vi "MGI RWA Process Array Elements.vi"(5 "Read/Write Options":T1={"TS Fmt"="", "Int Fmt"="", "Delimiter"=","}, 7 "Format String (%#0.15f)":string="%#0.15f", 8 "Error In":errorcluster, 9 "Name In":string, 10 "Array Variant":variant, 11 "Queue In":refnum<queue>) -> (0 "Error Out":errorcluster, 1 "Data Out":string, 3 "Queue Out":refnum<queue>)   [LabVIEW 2024]
doc: "This VI was created for use with the Read/Write Anything VIs. It converts array elements of the cluster to strings to be written to file.\n\nAuthored by Robert C. Mortensen\nsupport@mooregoodideas.com\nwww.mooregoodideas.com\n\nCopyright (c) 2010, Moore Good Ideas, Inc.\n\nAll rights reserved.\n\nRedistribution and use in source and binary forms, with or without modification, are permitted provided that the following conditions are met:\n\n * Redistributions of source code must retain the above copyright notice, this list of conditions and the following disclaimer.\n * Redistributions in binary form must reproduce the above copyright notice, this list of conditions and the following disclaimer in the documentation and/or other materials provided with the distribution.\n * Neither the name of Moore Good Ideas, Inc. nor the names of its contributors may be used to endorse or promote products derived from this software without specific prior written permission.\n\nTHIS SOFTWARE IS PROVIDED BY THE COPYRIGHT HOLDERS AND CONTRIBUTORS \"AS IS\" AND ANY EXPRESS OR IMPLIED WARRANTIES, INCLUDING, BUT NOT LIMITED TO, THE IMPLIED WARRANTIES OF MERCHANTABILITY AND FITNESS FOR A PARTICULAR PURPOSE ARE DISCLAIMED. IN NO EVENT SHALL THE COPYRIGHT OWNER OR CONTRIBUTORS BE LIABLE FOR ANY DIRECT, INDIRECT, INCIDENTAL, SPECIAL, EXEMPLARY, OR CONSEQUENTIAL DAMAGES (INCLUDING, BUT NOT LIMITED TO, PROCUREMENT OF SUBSTITUTE GOODS OR SERVICES; LOSS OF USE, DATA, OR PROFITS; OR BUSINESS INTERRUPTION) HOWEVER CAUSED AND ON ANY THEORY OF LIABILITY, WHETHER IN CONTRACT, STRICT LIABILITY, OR TORT (INCLUDING NEGLIGENCE OR OTHERWISE) ARISING IN ANY WAY OUT OF THE USE OF THIS SOFTWARE, EVEN IF ADVISED OF THE POSSIBILITY OF SUCH DAMAGE."
uses:
  MGI RWA Options Cluster.ctl
  MGI RWA Convertion Direction Enum.ctl
  VariantType.lvlib
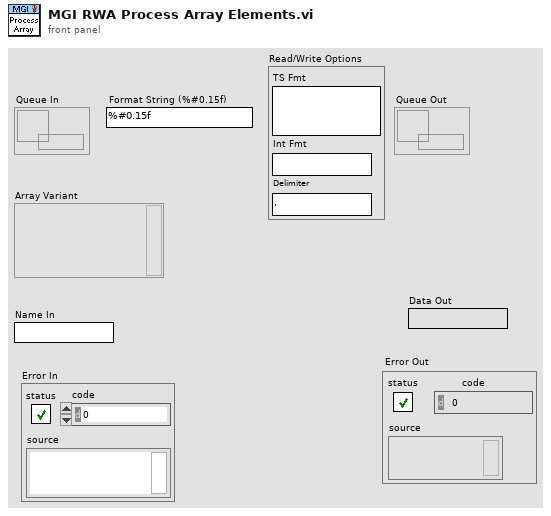
[diagram p1: front panel]
types:
  T1 = typedef "MGI RWA Options Cluster.ctl" = cluster{"TS Fmt":string, "Int Fmt":string, "Delimiter":string}
  T2 = typedef "VariantType.lvlib/Type.ctl" = enum8{"Invalid Type", "Void", "I8", "I16", "I32", "I64", "U8", "U16", "U32", "U64", "Single Float", "Double Float", "Extended Float", "Single Complex", "Double Complex", "Extended Complex", "Enum U8", "Enum U16", "Enum U32", "Enum U64", "Single Float With Unit", "Double Float With Unit", "Extended Float With Unit", "Single Complex with Unit", "Double Complex with Unit", "Extended Complex with Unit", "Boolean", "String", "Path", "Picture", "Tag", "Array", "Cluster", "Variant", "LV Variant", "Waveform", "Timestamp", "Digital Waveform", "Digital Data", "ExpressData", "Refnum", "External Data", "VI", "Poly VI", "LabVIEW Class Instance", "Fixed Point"}
  T3 = typedef "MGI RWA Convertion Direction Enum.ctl" = enum16{"String->Anything", "Anything->String"}
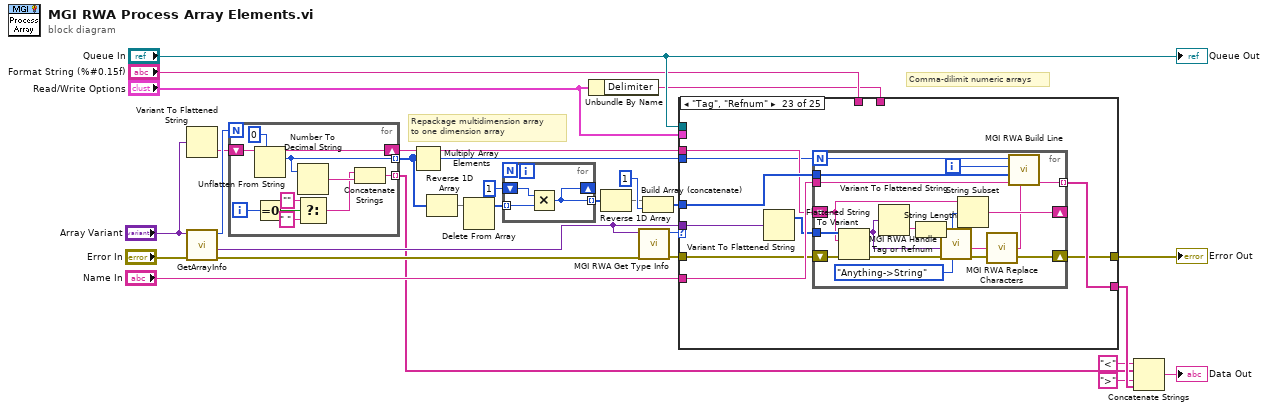
[diagram p0: block diagram]
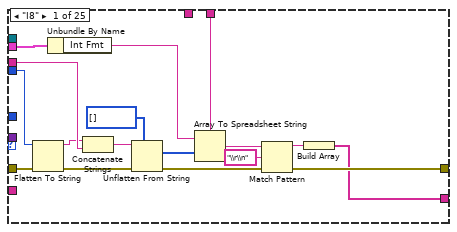
[diagram p2: hidden frame]
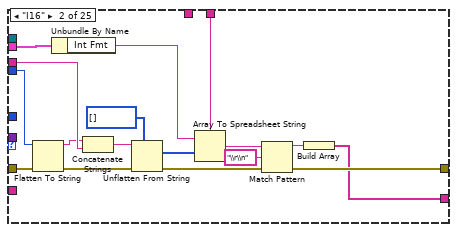
[diagram p3: hidden frame]
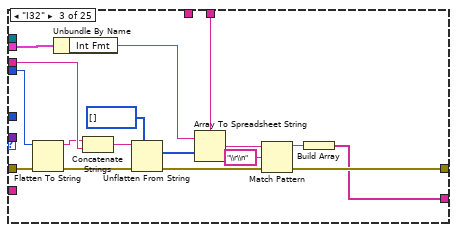
[diagram p4: hidden frame]
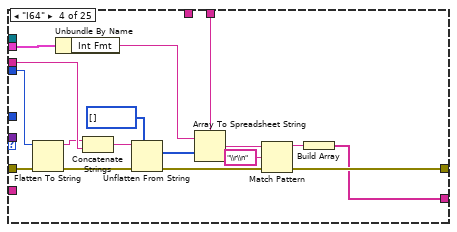
[diagram p5: hidden frame]
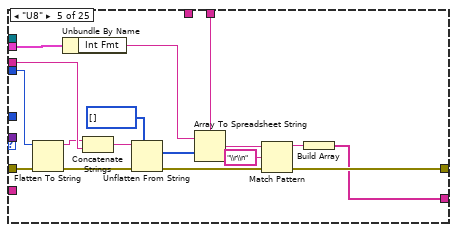
[diagram p6: hidden frame]
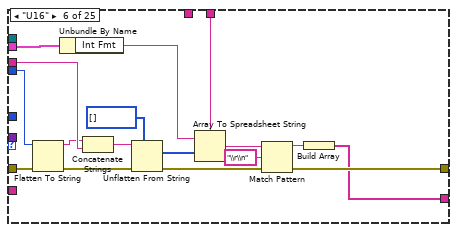
[diagram p7: hidden frame]
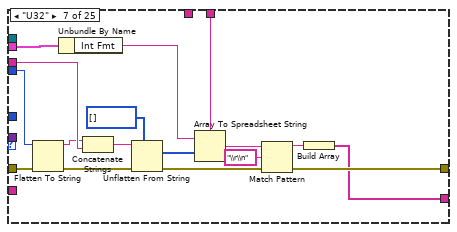
[diagram p8: hidden frame]
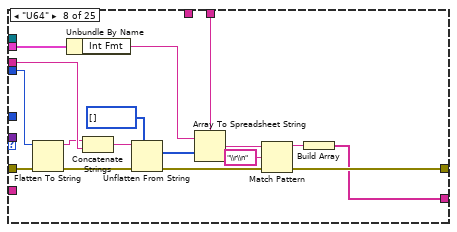
[diagram p9: hidden frame]
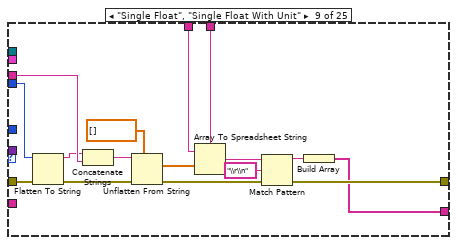
[diagram p10: hidden frame]
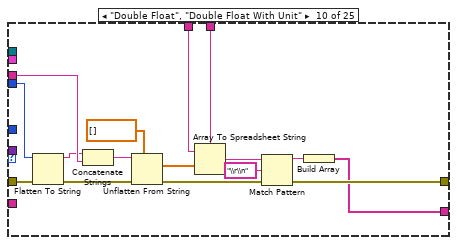
[diagram p11: hidden frame]
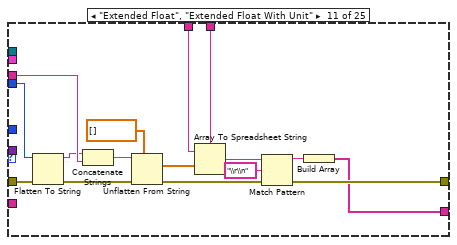
[diagram p12: hidden frame]
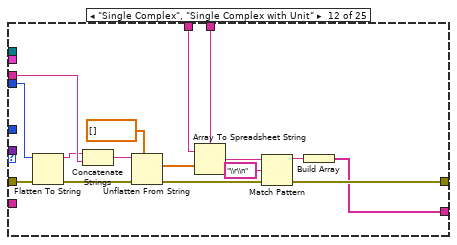
[diagram p13: hidden frame]
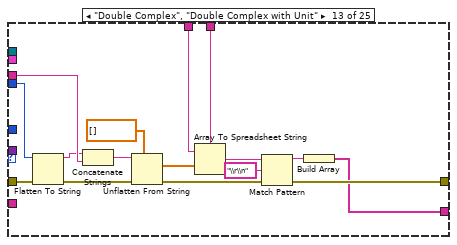
[diagram p14: hidden frame]
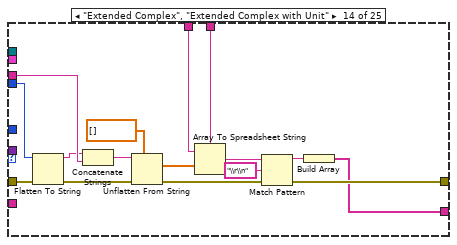
[diagram p15: hidden frame]
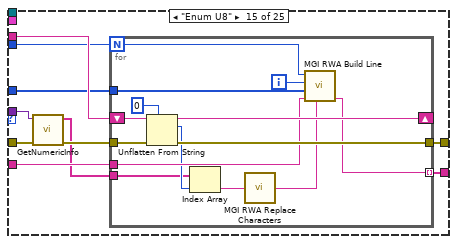
[diagram p16: hidden frame]
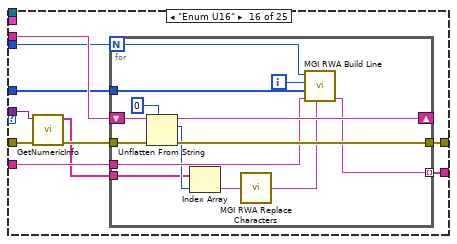
[diagram p17: hidden frame]
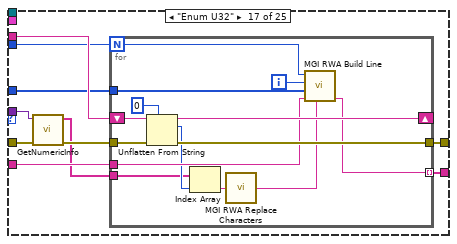
[diagram p18: hidden frame]
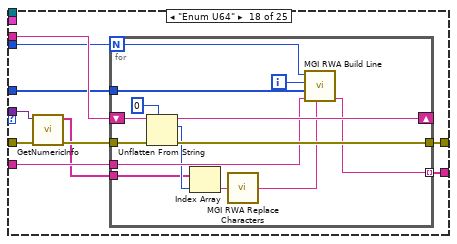
[diagram p19: hidden frame]
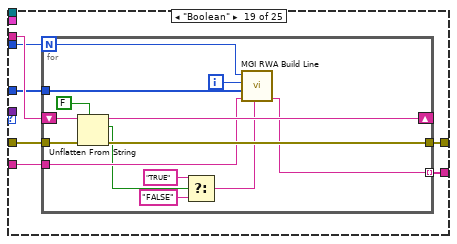
[diagram p20: hidden frame]
diagram:
  # "Comma-dilimit numeric arrays"
  # "Repackage multidimension array\nto one dimension array"
  n1 = Variant To Flattened String(Variant="Array Variant") -> (data string=w26:string)  [unwired: 1 out]
  n2 = call "GetArrayInfo.vi"("error in (no error)"="Error In", "Variant"="Array Variant") -> ("error out"=w8:errorcluster, "ArrayElement"=w9:variant, "NDims"=w27:i32)  [unwired: 6 in, 1 out]
  n3 = for {
    N: w27 -> [_]
    shift-right: [w38] -> w24
    shift-left: w26 -> [w39]
    tunnel: [w35] -> w13 mode=indexing
    tunnel: [w36] -> w7 mode=indexing
    i -> [w34]
    n4 = Unflatten From String(type=u32 0, binary string=w39) -> (rest of the binary string=w38:string, value=w35:u32)  [unwired: 3 in, 1 out]
    n5 = Equal To 0?(x=w34) -> (x = 0?=w33:bool)
    n6 = Number To Decimal String(number=w35) -> (decimal integer string=w37:string)  [unwired: 1 in]
    n7 = Select(t="", s=w33, f=" ") -> (s? t:f=w31:string)
    n8 = Concatenate Strings(w31, w37) -> (w36:string)
  }
  n9 = Multiply Array Elements(1:w13) -> (0:w23:u32)
  n10 = Reverse 1D Array(array=w13) -> (reversed array=w14:u32[])
  n11 = Delete From Array(array=w14) -> (array with subset deleted=w15:u32[])  [unwired: 2 in, 1 out]
  n12 = for {
    tunnel: w15 -> [w43] mode=indexing
    shift-right: [w41] -> _
    shift-left: i8 1 -> [w42]
    tunnel: [w41] -> w17 mode=indexing
    n13 = Multiply(x=w42, y=w43) -> (x*y=w41:u32)
  }
  n14 = Unbundle By Name("Read/Write Options") -> ("Delimiter"=w1:string)
  n15 = Reverse 1D Array(array=w17) -> (reversed array=w18:u32[])
  n16 = call "MGI RWA Get Type Info.vi"("Error In"=w8, "Variant"=w9) -> ("Error Out"=w25:errorcluster, "Type Enum"=w4:T2)  [unwired: 7 in, 1 out]
  n17 = Build Array (concatenate)(w18, i8 1) -> (w12:u32[])
  n18 = case shown="\"Tag\", \"Refnum\"" w4 {
    tunnel: [w59 w75 w91 w107 w123 w139 w155 w171 w186 w201 w216 w231 w246 w261 w271 w295 w319 w343 w364 w385 w404 w427 w462 w487 w497] -> w11
    tunnel: w25 -> [w48 w64 w80 w96 w112 w128 w144 w160 w175 w190 w205 w220 w235 w250 w264 w288 w312 w336 w363 w384 w403 w426 w461 w487 w505]
    tunnel: w24 -> [w58 w74 w90 w106 w122 w138 w154 w170 w185 w200 w215 w230 w245 w260 w270 w294 w318 w342 w362 w383 w402 w425 w464 w486 w492]
    tunnel: w23 -> [w57 w73 w89 w105 w121 w137 w153 w169 w184 w199 w214 w229 w244 w259 w269 w293 w317 w341 w361 w382 w401 w424 w463 _ w504]
    tunnel: "Name In" -> [_ _ _ _ _ _ _ _ _ _ _ _ _ _ w268 w292 w316 w340 w360 w381 w400 w423 w467 _ w503]
    tunnel: [w56 w72 w88 w104 w120 w136 w152 w168 w183 w198 w213 w228 w243 w258 w266 w290 w314 w338 w358 w379 w398 w421 w465 w485 _] -> w21
    tunnel: w12 -> [_ _ _ _ _ _ _ _ _ _ _ _ _ _ w267 w291 w315 w339 w359 w380 w399 w422 w466 _ w502]
    tunnel: "Queue In" -> [_ _ _ _ _ _ _ _ _ _ _ _ _ _ _ _ _ _ _ _ _ _ _ _ w498]
    tunnel: w9 -> [_ _ _ _ _ _ _ _ _ _ _ _ _ _ w265 w289 w313 w337 _ _ _ _ w460 _ w495]
    tunnel: "Format String (%#0.15f)" -> [_ _ _ _ _ _ _ _ w173 w188 w203 w218 w233 w248 _ _ _ _ _ _ _ _ _ _ _]
    tunnel: w1 -> [w46 w62 w78 w94 w110 w126 w142 w158 w172 w187 w202 w217 w232 w247 _ _ _ _ _ _ _ _ _ _ _]
    tunnel: "Read/Write Options" -> [w45 w61 w77 w93 w109 w125 w141 w157 _ _ _ _ _ _ _ _ _ _ _ _ _ w420 _ _ _]
    frame "I8" {
      n19 = Flatten To String(anything=w57, error in (no error)=w48) -> (data string=w53:string, error out=w47:errorcluster)  [unwired: 2 in, 1 out]
      n20 = Unbundle By Name(w45) -> ("Int Fmt"=w44:string)
      n21 = Concatenate Strings(w53, w58) -> (w54:string)
      n22 = Unflatten From String(type=i8[] [], binary string=w54, error in (no error)=w47) -> (value=w50:i8[], error out=w59:errorcluster)  [unwired: 2 in, 1 out]
      n23 = Array To Spreadsheet String(delimiter (Tab)=w46, array=w50, 3:w44) -> (spreadsheet string=w52:string)
      n24 = Match Pattern(string=w52, regular expression="\\r\\n") -> (before substring=w49:string)  [unwired: 1 in, 3 out]
      n25 = Build Array(w49) -> (w56:string[])
    }
    frame "I16" {
      n26 = Flatten To String(anything=w73, error in (no error)=w64) -> (data string=w69:string, error out=w63:errorcluster)  [unwired: 2 in, 1 out]
      n27 = Unbundle By Name(w61) -> ("Int Fmt"=w60:string)
      n28 = Concatenate Strings(w69, w74) -> (w70:string)
      n29 = Unflatten From String(type=i16[] [], binary string=w70, error in (no error)=w63) -> (value=w66:i16[], error out=w75:errorcluster)  [unwired: 2 in, 1 out]
      n30 = Array To Spreadsheet String(delimiter (Tab)=w62, array=w66, 3:w60) -> (spreadsheet string=w68:string)
      n31 = Match Pattern(string=w68, regular expression="\\r\\n") -> (before substring=w65:string)  [unwired: 1 in, 3 out]
      n32 = Build Array(w65) -> (w72:string[])
    }
    frame "I32" {
      n33 = Flatten To String(anything=w89, error in (no error)=w80) -> (data string=w85:string, error out=w79:errorcluster)  [unwired: 2 in, 1 out]
      n34 = Unbundle By Name(w77) -> ("Int Fmt"=w76:string)
      n35 = Concatenate Strings(w85, w90) -> (w86:string)
      n36 = Unflatten From String(type=i32[] [], binary string=w86, error in (no error)=w79) -> (value=w82:i32[], error out=w91:errorcluster)  [unwired: 2 in, 1 out]
      n37 = Array To Spreadsheet String(delimiter (Tab)=w78, array=w82, 3:w76) -> (spreadsheet string=w84:string)
      n38 = Match Pattern(string=w84, regular expression="\\r\\n") -> (before substring=w81:string)  [unwired: 1 in, 3 out]
      n39 = Build Array(w81) -> (w88:string[])
    }
    frame "I64" {
      n40 = Flatten To String(anything=w105, error in (no error)=w96) -> (data string=w101:string, error out=w95:errorcluster)  [unwired: 2 in, 1 out]
      n41 = Unbundle By Name(w93) -> ("Int Fmt"=w92:string)
      n42 = Concatenate Strings(w101, w106) -> (w102:string)
      n43 = Unflatten From String(type=i64[] [], binary string=w102, error in (no error)=w95) -> (value=w98:i64[], error out=w107:errorcluster)  [unwired: 2 in, 1 out]
      n44 = Array To Spreadsheet String(delimiter (Tab)=w94, array=w98, 3:w92) -> (spreadsheet string=w100:string)
      n45 = Match Pattern(string=w100, regular expression="\\r\\n") -> (before substring=w97:string)  [unwired: 1 in, 3 out]
      n46 = Build Array(w97) -> (w104:string[])
    }
    frame "U8" {
      n47 = Flatten To String(anything=w121, error in (no error)=w112) -> (data string=w117:string, error out=w111:errorcluster)  [unwired: 2 in, 1 out]
      n48 = Unbundle By Name(w109) -> ("Int Fmt"=w108:string)
      n49 = Concatenate Strings(w117, w122) -> (w118:string)
      n50 = Unflatten From String(type=u8[] [], binary string=w118, error in (no error)=w111) -> (value=w114:u8[], error out=w123:errorcluster)  [unwired: 2 in, 1 out]
      n51 = Array To Spreadsheet String(delimiter (Tab)=w110, array=w114, 3:w108) -> (spreadsheet string=w116:string)
      n52 = Match Pattern(string=w116, regular expression="\\r\\n") -> (before substring=w113:string)  [unwired: 1 in, 3 out]
      n53 = Build Array(w113) -> (w120:string[])
    }
    frame "U16" {
      n54 = Flatten To String(anything=w137, error in (no error)=w128) -> (data string=w133:string, error out=w127:errorcluster)  [unwired: 2 in, 1 out]
      n55 = Unbundle By Name(w125) -> ("Int Fmt"=w124:string)
      n56 = Concatenate Strings(w133, w138) -> (w134:string)
      n57 = Unflatten From String(type=u16[] [], binary string=w134, error in (no error)=w127) -> (value=w130:u16[], error out=w139:errorcluster)  [unwired: 2 in, 1 out]
      n58 = Array To Spreadsheet String(delimiter (Tab)=w126, array=w130, 3:w124) -> (spreadsheet string=w132:string)
      n59 = Match Pattern(string=w132, regular expression="\\r\\n") -> (before substring=w129:string)  [unwired: 1 in, 3 out]
      n60 = Build Array(w129) -> (w136:string[])
    }
    frame "U32" {
      n61 = Flatten To String(anything=w153, error in (no error)=w144) -> (data string=w149:string, error out=w143:errorcluster)  [unwired: 2 in, 1 out]
      n62 = Unbundle By Name(w141) -> ("Int Fmt"=w140:string)
      n63 = Concatenate Strings(w149, w154) -> (w150:string)
      n64 = Unflatten From String(type=u32[] [], binary string=w150, error in (no error)=w143) -> (value=w146:u32[], error out=w155:errorcluster)  [unwired: 2 in, 1 out]
      n65 = Array To Spreadsheet String(delimiter (Tab)=w142, array=w146, 3:w140) -> (spreadsheet string=w148:string)
      n66 = Match Pattern(string=w148, regular expression="\\r\\n") -> (before substring=w145:string)  [unwired: 1 in, 3 out]
      n67 = Build Array(w145) -> (w152:string[])
    }
    frame "U64" {
      n68 = Flatten To String(anything=w169, error in (no error)=w160) -> (data string=w165:string, error out=w159:errorcluster)  [unwired: 2 in, 1 out]
      n69 = Unbundle By Name(w157) -> ("Int Fmt"=w156:string)
      n70 = Concatenate Strings(w165, w170) -> (w166:string)
      n71 = Unflatten From String(type=u64[] [], binary string=w166, error in (no error)=w159) -> (value=w162:u64[], error out=w171:errorcluster)  [unwired: 2 in, 1 out]
      n72 = Array To Spreadsheet String(delimiter (Tab)=w158, array=w162, 3:w156) -> (spreadsheet string=w164:string)
      n73 = Match Pattern(string=w164, regular expression="\\r\\n") -> (before substring=w161:string)  [unwired: 1 in, 3 out]
      n74 = Build Array(w161) -> (w168:string[])
    }
    frame "Single Float", "Single Float With Unit" {
      n75 = Flatten To String(anything=w184, error in (no error)=w175) -> (data string=w180:string, error out=w174:errorcluster)  [unwired: 2 in, 1 out]
      n76 = Concatenate Strings(w180, w185) -> (w181:string)
      n77 = Unflatten From String(type=sgl[] [], binary string=w181, error in (no error)=w174) -> (value=w177:sgl[], error out=w186:errorcluster)  [unwired: 2 in, 1 out]
      n78 = Array To Spreadsheet String(delimiter (Tab)=w172, array=w177, 3:w173) -> (spreadsheet string=w179:string)
      n79 = Match Pattern(string=w179, regular expression="\\r\\n") -> (before substring=w176:string)  [unwired: 1 in, 3 out]
      n80 = Build Array(w176) -> (w183:string[])
    }
    frame "Double Float", "Double Float With Unit" {
      n81 = Flatten To String(anything=w199, error in (no error)=w190) -> (data string=w195:string, error out=w189:errorcluster)  [unwired: 2 in, 1 out]
      n82 = Concatenate Strings(w195, w200) -> (w196:string)
      n83 = Unflatten From String(type=dbl[] [], binary string=w196, error in (no error)=w189) -> (value=w192:dbl[], error out=w201:errorcluster)  [unwired: 2 in, 1 out]
      n84 = Array To Spreadsheet String(delimiter (Tab)=w187, array=w192, 3:w188) -> (spreadsheet string=w194:string)
      n85 = Match Pattern(string=w194, regular expression="\\r\\n") -> (before substring=w191:string)  [unwired: 1 in, 3 out]
      n86 = Build Array(w191) -> (w198:string[])
    }
    frame "Extended Float", "Extended Float With Unit" {
      n87 = Flatten To String(anything=w214, error in (no error)=w205) -> (data string=w210:string, error out=w204:errorcluster)  [unwired: 2 in, 1 out]
      n88 = Concatenate Strings(w210, w215) -> (w211:string)
      n89 = Unflatten From String(type=ext[] [], binary string=w211, error in (no error)=w204) -> (value=w207:ext[], error out=w216:errorcluster)  [unwired: 2 in, 1 out]
      n90 = Array To Spreadsheet String(delimiter (Tab)=w202, array=w207, 3:w203) -> (spreadsheet string=w209:string)
      n91 = Match Pattern(string=w209, regular expression="\\r\\n") -> (before substring=w206:string)  [unwired: 1 in, 3 out]
      n92 = Build Array(w206) -> (w213:string[])
    }
    frame "Single Complex", "Single Complex with Unit" {
      n93 = Flatten To String(anything=w229, error in (no error)=w220) -> (data string=w225:string, error out=w219:errorcluster)  [unwired: 2 in, 1 out]
      n94 = Concatenate Strings(w225, w230) -> (w226:string)
      n95 = Unflatten From String(type=csg[] [], binary string=w226, error in (no error)=w219) -> (value=w222:csg[], error out=w231:errorcluster)  [unwired: 2 in, 1 out]
      n96 = Array To Spreadsheet String(delimiter (Tab)=w217, array=w222, 3:w218) -> (spreadsheet string=w224:string)
      n97 = Match Pattern(string=w224, regular expression="\\r\\n") -> (before substring=w221:string)  [unwired: 1 in, 3 out]
      n98 = Build Array(w221) -> (w228:string[])
    }
    frame "Double Complex", "Double Complex with Unit" {
      n99 = Flatten To String(anything=w244, error in (no error)=w235) -> (data string=w240:string, error out=w234:errorcluster)  [unwired: 2 in, 1 out]
      n100 = Concatenate Strings(w240, w245) -> (w241:string)
      n101 = Unflatten From String(type=cdb[] [], binary string=w241, error in (no error)=w234) -> (value=w237:cdb[], error out=w246:errorcluster)  [unwired: 2 in, 1 out]
      n102 = Array To Spreadsheet String(delimiter (Tab)=w232, array=w237, 3:w233) -> (spreadsheet string=w239:string)
      n103 = Match Pattern(string=w239, regular expression="\\r\\n") -> (before substring=w236:string)  [unwired: 1 in, 3 out]
      n104 = Build Array(w236) -> (w243:string[])
    }
    frame "Extended Complex", "Extended Complex with Unit" {
      n105 = Flatten To String(anything=w259, error in (no error)=w250) -> (data string=w255:string, error out=w249:errorcluster)  [unwired: 2 in, 1 out]
      n106 = Concatenate Strings(w255, w260) -> (w256:string)
      n107 = Unflatten From String(type=cxt[] [], binary string=w256, error in (no error)=w249) -> (value=w252:cxt[], error out=w261:errorcluster)  [unwired: 2 in, 1 out]
      n108 = Array To Spreadsheet String(delimiter (Tab)=w247, array=w252, 3:w248) -> (spreadsheet string=w254:string)
      n109 = Match Pattern(string=w254, regular expression="\\r\\n") -> (before substring=w251:string)  [unwired: 1 in, 3 out]
      n110 = Build Array(w251) -> (w258:string[])
    }
    frame "Enum U8" {
      n111 = call "GetNumericInfo.vi"("error in (no error)"=w264, "Variant"=w265) -> ("error out"=w263:errorcluster, "EnumNames"=w262:string[])  [unwired: 6 in, 2 out]
      n112 = for {
        N: w269 -> [w281]
        tunnel: [w282] -> w271
        tunnel: w263 -> [w283]
        shift-right: [w284] -> _
        shift-left: w270 -> [w285]
        tunnel: w268 -> [w277]
        tunnel: [w278] -> w266 mode=indexing
        tunnel: w267 -> [w279]
        tunnel: w262 -> [w274]
        i -> [w280]
        n113 = Unflatten From String(type=u8 0, binary string=w285, error in (no error)=w283) -> (rest of the binary string=w284:string, value=w275:u8, error out=w282:errorcluster)  [unwired: 2 in]
        n114 = Index Array(array=w274, index=w275) -> (element=w273:string)
        n115 = call "MGI RWA Replace Characters.vi"("String In"=w273) -> ("String Out"=w272:string)  [unwired: 1 in]
        n116 = call "MGI RWA Build Line.vi"("Value String (\"\")"=w272, "Name In"=w277, "Array"=w279, "Iteration"=w280, "Iterations"=w281) -> ("Line"=w278:string)  [unwired: 5 in, 1 out]
      }
    }
    frame "Enum U16" {
      n117 = call "GetNumericInfo.vi"("error in (no error)"=w288, "Variant"=w289) -> ("error out"=w287:errorcluster, "EnumNames"=w286:string[])  [unwired: 6 in, 2 out]
      n118 = for {
        N: w293 -> [w305]
        tunnel: [w306] -> w295
        tunnel: w287 -> [w307]
        shift-right: [w308] -> _
        shift-left: w294 -> [w309]
        tunnel: w292 -> [w301]
        tunnel: [w302] -> w290 mode=indexing
        tunnel: w291 -> [w303]
        tunnel: w286 -> [w298]
        i -> [w304]
        n119 = Unflatten From String(type=u16 0, binary string=w309, error in (no error)=w307) -> (rest of the binary string=w308:string, value=w299:u16, error out=w306:errorcluster)  [unwired: 2 in]
        n120 = Index Array(array=w298, index=w299) -> (element=w297:string)
        n121 = call "MGI RWA Replace Characters.vi"("String In"=w297) -> ("String Out"=w296:string)  [unwired: 1 in]
        n122 = call "MGI RWA Build Line.vi"("Value String (\"\")"=w296, "Name In"=w301, "Array"=w303, "Iteration"=w304, "Iterations"=w305) -> ("Line"=w302:string)  [unwired: 5 in, 1 out]
      }
    }
    frame "Enum U32" {
      n123 = call "GetNumericInfo.vi"("error in (no error)"=w312, "Variant"=w313) -> ("error out"=w311:errorcluster, "EnumNames"=w310:string[])  [unwired: 6 in, 2 out]
      n124 = for {
        N: w317 -> [w329]
        tunnel: [w330] -> w319
        tunnel: w311 -> [w331]
        shift-right: [w332] -> _
        shift-left: w318 -> [w333]
        tunnel: w316 -> [w325]
        tunnel: [w326] -> w314 mode=indexing
        tunnel: w315 -> [w327]
        tunnel: w310 -> [w322]
        i -> [w328]
        n125 = Unflatten From String(type=u32 0, binary string=w333, error in (no error)=w331) -> (rest of the binary string=w332:string, value=w323:u32, error out=w330:errorcluster)  [unwired: 2 in]
        n126 = Index Array(array=w322, index=w323) -> (element=w321:string)
        n127 = call "MGI RWA Replace Characters.vi"("String In"=w321) -> ("String Out"=w320:string)  [unwired: 1 in]
        n128 = call "MGI RWA Build Line.vi"("Value String (\"\")"=w320, "Name In"=w325, "Array"=w327, "Iteration"=w328, "Iterations"=w329) -> ("Line"=w326:string)  [unwired: 5 in, 1 out]
      }
    }
    frame "Enum U64" {
      n129 = call "GetNumericInfo.vi"("error in (no error)"=w336, "Variant"=w337) -> ("error out"=w335:errorcluster, "EnumNames"=w334:string[])  [unwired: 6 in, 2 out]
      n130 = for {
        N: w341 -> [w353]
        tunnel: [w354] -> w343
        tunnel: w335 -> [w355]
        shift-right: [w356] -> _
        shift-left: w342 -> [w357]
        tunnel: w340 -> [w349]
        tunnel: [w350] -> w338 mode=indexing
        tunnel: w339 -> [w351]
        tunnel: w334 -> [w346]
        i -> [w352]
        n131 = Unflatten From String(type=u64 0, binary string=w357, error in (no error)=w355) -> (rest of the binary string=w356:string, value=w347:u64, error out=w354:errorcluster)  [unwired: 2 in]
        n132 = Index Array(array=w346, index=w347) -> (element=w345:string)
        n133 = call "MGI RWA Replace Characters.vi"("String In"=w345) -> ("String Out"=w344:string)  [unwired: 1 in]
        n134 = call "MGI RWA Build Line.vi"("Value String (\"\")"=w344, "Name In"=w349, "Array"=w351, "Iteration"=w352, "Iterations"=w353) -> ("Line"=w350:string)  [unwired: 5 in, 1 out]
      }
    }
    frame "Boolean" {
      n135 = for {
        N: w361 -> [w374]
        tunnel: [w375] -> w364
        tunnel: w363 -> [w376]
        shift-right: [w377] -> _
        shift-left: w362 -> [w378]
        tunnel: w360 -> [w370]
        tunnel: [w371] -> w358 mode=indexing
        tunnel: w359 -> [w372]
        i -> [w373]
        n136 = Unflatten From String(type=FALSE, binary string=w378, error in (no error)=w376) -> (rest of the binary string=w377:string, value=w366:bool, error out=w375:errorcluster)  [unwired: 2 in]
        n137 = Select(t="TRUE", s=w366, f="FALSE") -> (s? t:f=w365:string)
        n138 = call "MGI RWA Build Line.vi"("Value String (\"\")"=w365, "Name In"=w370, "Array"=w372, "Iteration"=w373, "Iterations"=w374) -> ("Line"=w371:string)  [unwired: 5 in, 1 out]
      }
    }
    frame "String" {
      n139 = for {
        N: w382 -> [w393]
        tunnel: [w394] -> w385
        tunnel: w384 -> [w395]
        shift-right: [w396] -> _
        shift-left: w383 -> [w397]
        tunnel: w381 -> [w389]
        tunnel: [w390] -> w379 mode=indexing
        tunnel: w380 -> [w391]
        i -> [w392]
        n140 = Unflatten From String(type="", binary string=w397, error in (no error)=w395) -> (rest of the binary string=w396:string, value=w387:string, error out=w394:errorcluster)  [unwired: 2 in]
        n141 = call "MGI RWA Replace Characters.vi"("String In"=w387) -> ("String Out"=w386:string)  [unwired: 1 in]
        n142 = call "MGI RWA Build Line.vi"("Value String (\"\")"=w386, "Name In"=w389, "Array"=w391, "Iteration"=w392, "Iterations"=w393) -> ("Line"=w390:string)  [unwired: 5 in, 1 out]
      }
    }
    frame "Path" {
      n143 = for {
        N: w401 -> [w413]
        tunnel: [w414] -> w404
        tunnel: w403 -> [w415]
        shift-right: [w416] -> _
        shift-left: w402 -> [w417]
        tunnel: w400 -> [w409]
        tunnel: [w410] -> w398 mode=indexing
        tunnel: w399 -> [w411]
        i -> [w412]
        n144 = Unflatten From String(type=path "", binary string=w417, error in (no error)=w415) -> (rest of the binary string=w416:string, value=w407:path, error out=w414:errorcluster)  [unwired: 2 in]
        n145 = Path To String(path=w407) -> (string=w406:string)
        n146 = call "MGI RWA Replace Characters.vi"("String In"=w406) -> ("String Out"=w405:string)  [unwired: 1 in]
        n147 = call "MGI RWA Build Line.vi"("Value String (\"\")"=w405, "Name In"=w409, "Array"=w411, "Iteration"=w412, "Iterations"=w413) -> ("Line"=w410:string)  [unwired: 5 in, 1 out]
      }
    }
    frame "Timestamp" {
      n148 = Unbundle By Name(w420) -> ("TS Fmt"=w419:string)
      n149 = for {
        N: w424 -> [w435]
        tunnel: [w436] -> w427
        tunnel: w426 -> [w437]
        shift-right: [w438] -> _
        shift-left: w425 -> [w439]
        tunnel: w423 -> [w432]
        tunnel: [w433] -> w421 mode=indexing
        tunnel: w422 -> [w434]
        tunnel: w419 -> [w429]
        tunnel: timestamp(0 s since 1904-01-01) -> [w430]
        i -> [w428]
        n150 = case shown="\"\"" w429 {
          selector: w429 -> [_ w450]
          tunnel: w439 -> [w445 w458]
          tunnel: [w445 w457] -> w438
          tunnel: w437 -> [w448 w456]
          tunnel: [w448 w455] -> w436
          tunnel: [w440 w454] -> w431
          tunnel: w430 -> [_ w452]
          tunnel: w428 -> [w449 _]
          frame "" {
            w446 = 16 ("y")
            n151 = Multiply(x=w449, y=w446) -> (x*y=w447:i32)
            n152 = String Subset(string=w445, offset (0)=w447, length (rest)=w446) -> (substring=w441:string)
            n153 = String To Byte Array(string=w441) -> (unsigned byte array=w443:u8[])
            n154 = call "MGI U8 Data to Hex Str.vi"("u8 Data[]"=w443) -> ("HEX String (0-9,A-F)"=w444:string)
            n155 = Concatenate Strings("0x", w444) -> (w440:string)
          }
          frame Default {
            n156 = Unflatten From String(type=w452, binary string=w458, error in (no error)=w456) -> (rest of the binary string=w457:string, value=w453:timestamp, error out=w455:errorcluster)  [unwired: 2 in]
            n157 = Format Date/Time String(time format string (%c)=w450, seconds (now)=w453) -> (date/time string=w451:string)  [unwired: 1 in]
            n158 = call "MGI RWA Replace Characters.vi"("String In"=w451) -> ("String Out"=w454:string)  [unwired: 1 in]
          }
        }
        n159 = call "MGI RWA Build Line.vi"("Value String (\"\")"=w431, "Name In"=w432, "Array"=w434, "Iteration"=w428, "Iterations"=w435) -> ("Line"=w433:string)  [unwired: 5 in, 1 out]
      }
    }
    frame "Tag", "Refnum" {
      n160 = Variant To Flattened String(Variant=w460) -> (1:w459:i16[])  [unwired: 1 out]
      n161 = for {
        N: w463 -> [w484]
        tunnel: w467 -> [w478]
        tunnel: w466 -> [w482]
        tunnel: w459 -> [w480]
        shift-right: [w475] -> _
        shift-left: w464 -> [w476]
        tunnel: [w474] -> w465 mode=indexing
        shift-right: [w471] -> w462
        shift-left: w461 -> [w481]
        i -> [w483]
        n162 = Flattened String To Variant(4:w481, 6:w476, 7:w480) -> (0:w472:errorcluster, 3:w473:variant)
        n163 = Variant To Flattened String(Variant=w473) -> (data string=w479:string)  [unwired: 1 out]
        n164 = String Length(string=w479) -> (length=w477:i32)
        n165 = call "MGI RWA Handle Tag or Refnum.vi"("Conversion"=MGI_RWA_Convertion_Direction_Enum."Anything->String", "Error In"=w472, "Anything"=w473) -> ("Error Out"=w471:errorcluster, "String"=w470:string)  [unwired: 7 in]
        n166 = String Subset(string=w476, offset (0)=w477) -> (substring=w475:string)  [unwired: 1 in]
        n167 = call "MGI RWA Replace Characters.vi"("String In"=w470) -> ("String Out"=w469:string)  [unwired: 1 in]
        n168 = call "MGI RWA Build Line.vi"("Value String (\"\")"=w469, "Name In"=w478, "Array"=w482, "Iteration"=w483, "Iterations"=w484) -> ("Line"=w474:string)  [unwired: 5 in, 1 out]
      }
    }
    frame Default {
      n169 = String To Byte Array(string=w486) -> (unsigned byte array=w491:u8[])
      n170 = Number To Hexadecimal String(1:i16 2 ("width (-)"), 2:w491) -> (0:w490:string[])
      n171 = Build Array (concatenate)("0x", w490) -> (w485:string[])
    }
    frame "Cluster" {
      # "Enqueue cluster\nelements"
      n172 = Variant To Flattened String(Variant=w495) -> (1:w494:i16[])  [unwired: 1 out]
      n173 = for {
        N: w504 -> [w524]
        tunnel: [w518] -> w499
        tunnel: w505 -> [w520]
        tunnel: w503 -> [w515]
        tunnel: w502 -> [w522]
        tunnel: [w516] -> w500 mode=indexing
        tunnel: [w521] -> w496 mode=indexing
        tunnel: w494 -> [w519]
        shift-right: [w512] -> _
        shift-left: w492 -> [w513]
        i -> [w523]
        n174 = Flattened String To Variant(4:w520, 6:w513, 7:w519) -> (0:w518:errorcluster, 3:w516:variant)
        n175 = Variant To Flattened String(Variant=w516) -> (data string=w517:string)  [unwired: 1 out]
        n176 = String Length(string=w517) -> (length=w514:i32)
        n177 = String Subset(string=w513, offset (0)=w514) -> (substring=w512:string)  [unwired: 1 in]
        n178 = call "MGI RWA Build Line.vi"("Name In"=w515, "Array"=w522, "Iteration"=w523, "Iterations"=w524) -> ("Name Out"=w521:string)  [unwired: 6 in, 1 out]
      }
      n179 = Reverse 1D Array(array=w496) -> (reversed array=w493:string[])
      n180 = Reverse 1D Array(array=w500) -> (reversed array=w501:variant[])
      n181 = for {
        tunnel: [w511] -> w497
        tunnel: w501 -> [w510] mode=indexing
        tunnel: w499 -> [w509]
        tunnel: w498 -> [w507]
        tunnel: w493 -> [w506] mode=indexing
        n182 = Bundle("Variant"=w510, "Name Out"=w506) -> (w508:cluster{"Variant":variant, "Name Out":string})  [unwired: 1 in]
        n183 = Enqueue Element At Opposite End(queue=w507, element=w508, error in (no error)=w509) -> (error out=w511:errorcluster)  [unwired: 1 in, 2 out]
      }
    }
  }
  "Error Out" <- w11
  n184 = Concatenate Strings("<", w7, ">", w21) -> (→"Data Out":string)
  "Queue Out" <- "Queue In"
